vi "VI Tree.vi"   [LabVIEW 2020]
uses:
  GPP.lvlib
panel:
  # "SEE DIAGRAM\nFOR VI TREE."
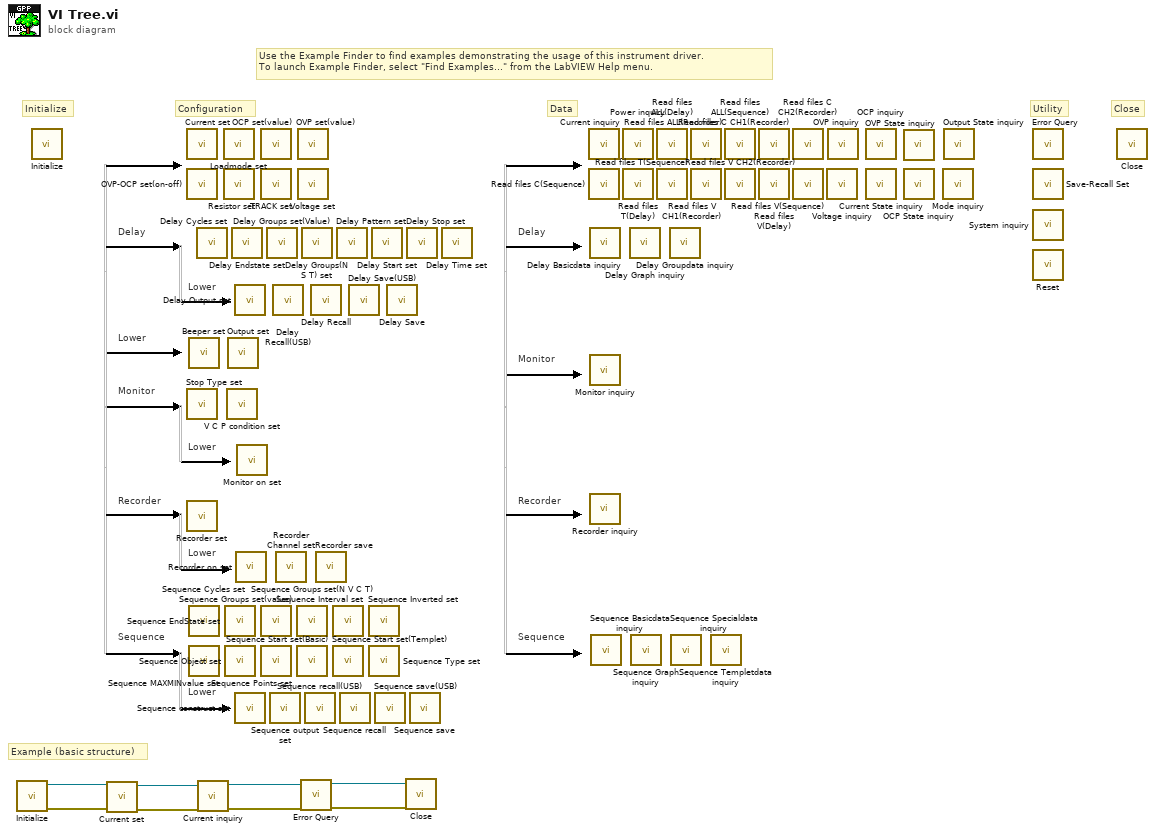
[diagram p0: block diagram]
diagram:
  # "Example (basic structure)"
  # "Sequence"
  # "Recorder"
  # "Monitor"
  # "Delay"
  # "Lower"
  # "Lower"
  # "Lower"
  # "Sequence"
  # "Recorder"
  # "Monitor"
  # "Lower"
  # "Lower"
  # "Delay"
  # "Configuration"
  # "Utility"
  # "Data"
  # "Close"
  # "Initialize"
  # "Use the Example Finder to find examples demonstrating the usage of this instrument driver.\nTo launch Example Finder, select \"Find Examples...\" from the LabVIEW Help menu."
  n1 = call "Initialize.vi"() -> ("error out"=w7:errorcluster, "VISA resource name out"=w8:refnum<visa-resource-name>)  [unwired: 9 in, 1 out]
  n2 = call "Initialize.vi"() -> ()  [unwired: 9 in, 3 out]
  n3 = call "Current set.vi"("error in (no error)"=w7, "VISA resource name"=w8) -> ("error out"=w5:errorcluster, "VISA resource name out"=w6:refnum<visa-resource-name>)  [unwired: 8 in]
  n4 = call "Current set.vi"() -> ()  [unwired: 10 in, 2 out]
  n5 = call "OVP-OCP set(on-off).vi"() -> ()  [unwired: 10 in, 2 out]
  n6 = call "Stop Type set.vi"() -> ()  [unwired: 10 in, 2 out]
  n7 = call "Recorder set.vi"() -> ()  [unwired: 10 in, 2 out]
  n8 = call "Beeper set.vi"() -> ()  [unwired: 10 in, 2 out]
  n9 = call "Sequence Cycles set.vi"() -> ()  [unwired: 10 in, 2 out]
  n10 = call "Sequence MAXMINvalue set.vi"() -> ()  [unwired: 10 in, 2 out]
  n11 = call "Delay Cycles set.vi"() -> ()  [unwired: 10 in, 2 out]
  n12 = call "Current inquiry.vi"("error in (no error)"=w5, "VISA resource name"=w6) -> ("error out"=w3:errorcluster, "VISA resource name out"=w4:refnum<visa-resource-name>)  [unwired: 7 in, 1 out]
  n13 = call "Loadmode set.vi"() -> ()  [unwired: 10 in, 2 out]
  n14 = call "Resistor set.vi"() -> ()  [unwired: 10 in, 2 out]
  n15 = call "Sequence EndState set.vi"() -> ()  [unwired: 10 in, 2 out]
  n16 = call "Sequence Object set.vi"() -> ()  [unwired: 10 in, 2 out]
  n17 = call "V C P condition set.vi"() -> ()  [unwired: 18 in, 2 out]
  n18 = call "Output set.vi"() -> ()  [unwired: 10 in, 2 out]
  n19 = call "Delay Endstate set.vi"() -> ()  [unwired: 10 in, 2 out]
  n20 = call "Delay Output set.vi"() -> ()  [unwired: 10 in, 2 out]
  n21 = call "Sequence construct set.vi"() -> ()  [unwired: 10 in, 2 out]
  n22 = call "Recorder on set.vi"() -> ()  [unwired: 10 in, 2 out]
  n23 = call "Monitor on set.vi"() -> ()  [unwired: 10 in, 2 out]
  n24 = call "OCP set(value).vi"() -> ()  [unwired: 10 in, 2 out]
  n25 = call "TRACK set.vi"() -> ()  [unwired: 10 in, 2 out]
  n26 = call "Sequence Groups set(value).vi"() -> ()  [unwired: 10 in, 2 out]
  n27 = call "Sequence Points set.vi"() -> ()  [unwired: 10 in, 2 out]
  n28 = call "Delay Groups set(Value).vi"() -> ()  [unwired: 10 in, 2 out]
  n29 = call "Sequence output set.vi"() -> ()  [unwired: 10 in, 2 out]
  n30 = call "Delay Recall(USB).vi"() -> ()  [unwired: 10 in, 2 out]
  n31 = call "Recorder Channel set.vi"() -> ()  [unwired: 10 in, 2 out]
  n32 = call "Sequence Groups set(N V C T).vi"() -> ()  [unwired: 10 in, 2 out]
  n33 = call "Sequence Start set(Basic).vi"() -> ()  [unwired: 10 in, 2 out]
  n34 = call "OVP set(value).vi"() -> ()  [unwired: 10 in, 2 out]
  n35 = call "Voltage set.vi"() -> ()  [unwired: 10 in, 2 out]
  n36 = call "Error Query.vi"("error in (no error)"=w3, "VISA resource name"=w4) -> ("error out"=w1:errorcluster, "VISA resource name out"=w2:refnum<visa-resource-name>)  [unwired: 6 in, 2 out]
  n37 = call "Delay Groups(N S T) set.vi"() -> ()  [unwired: 10 in, 2 out]
  n38 = call "Sequence recall(USB).vi"() -> ()  [unwired: 10 in, 2 out]
  n39 = call "Delay Recall.vi"() -> ()  [unwired: 10 in, 2 out]
  n40 = call "Recorder save.vi"() -> ()  [unwired: 10 in, 2 out]
  n41 = call "Sequence Interval set.vi"() -> ()  [unwired: 10 in, 2 out]
  n42 = call "Sequence Start set(Templet).vi"() -> ()  [unwired: 10 in, 2 out]
  n43 = call "Delay Pattern set.vi"() -> ()  [unwired: 10 in, 2 out]
  n44 = call "Sequence recall.vi"() -> ()  [unwired: 10 in, 2 out]
  n45 = call "Delay Save(USB).vi"() -> ()  [unwired: 10 in, 2 out]
  n46 = call "Sequence Inverted set.vi"() -> ()  [unwired: 10 in, 2 out]
  n47 = call "Sequence Type set.vi"() -> ()  [unwired: 10 in, 2 out]
  n48 = call "Delay Start set.vi"() -> ()  [unwired: 10 in, 2 out]
  n49 = call "Sequence save(USB).vi"() -> ()  [unwired: 10 in, 2 out]
  n50 = call "Delay Save.vi"() -> ()  [unwired: 10 in, 2 out]
  n51 = call "Close.vi"("error in (no error)"=w1, "VISA resource name"=w2) -> ()  [unwired: 9 in, 1 out]
  n52 = call "Delay Stop set.vi"() -> ()  [unwired: 10 in, 2 out]
  n53 = call "Sequence save.vi"() -> ()  [unwired: 10 in, 2 out]
  n54 = call "Delay Time set.vi"() -> ()  [unwired: 10 in, 2 out]
  n55 = call "Current inquiry.vi"() -> ()  [unwired: 9 in, 3 out]
  n56 = call "Read files C(Sequence).vi"() -> ()  [unwired: 11 in, 1 out]
  n57 = call "Delay Basicdata inquiry.vi"() -> ()  [unwired: 6 in, 6 out]
  n58 = call "Monitor inquiry.vi"() -> ()  [unwired: 7 in, 9 out]
  n59 = call "Recorder inquiry.vi"() -> ()  [unwired: 7 in, 5 out]
  n60 = call "Sequence Basicdata inquiry.vi"() -> ()  [unwired: 6 in, 6 out]
  n61 = call "Power inquiry.vi"() -> ()  [unwired: 9 in, 3 out]
  n62 = call "Read files T(Delay).vi"() -> ()  [unwired: 11 in, 1 out]
  n63 = call "Delay Graph inquiry.vi"() -> ()  [unwired: 12 in, 4 out]
  n64 = call "Sequence Graph inquiry.vi"() -> ()  [unwired: 12 in, 4 out]
  n65 = call "Read files ALL(Delay).vi"() -> ()  [unwired: 10 in, 2 out]
  n66 = call "Read files T(Sequence).vi"() -> ()  [unwired: 11 in, 1 out]
  n67 = call "Delay Groupdata inquiry.vi"() -> ()  [unwired: 8 in, 4 out]
  n68 = call "Sequence Specialdata inquiry.vi"() -> ()  [unwired: 6 in, 6 out]
  n69 = call "Read files ALL(Recorder).vi"() -> ()  [unwired: 8 in, 4 out]
  n70 = call "Read files V CH1(Recorder).vi"() -> ()  [unwired: 11 in, 1 out]
  n71 = call "Sequence Templetdata inquiry.vi"() -> ()  [unwired: 6 in, 10 out]
  n72 = call "Read files ALL(Sequence).vi"() -> ()  [unwired: 10 in, 2 out]
  n73 = call "Read files V CH2(Recorder).vi"() -> ()  [unwired: 11 in, 1 out]
  n74 = call "Read files C CH1(Recorder).vi"() -> ()  [unwired: 11 in, 1 out]
  n75 = call "Read files V(Delay).vi"() -> ()  [unwired: 11 in, 1 out]
  n76 = call "Read files C CH2(Recorder).vi"() -> ()  [unwired: 11 in, 1 out]
  n77 = call "Read files V(Sequence).vi"() -> ()  [unwired: 11 in, 1 out]
  n78 = call "Voltage inquiry.vi"() -> ()  [unwired: 9 in, 3 out]
  n79 = call "OVP inquiry.vi"() -> ()  [unwired: 9 in, 3 out]
  n80 = call "OCP inquiry.vi"() -> ()  [unwired: 9 in, 3 out]
  n81 = call "Current State inquiry.vi"() -> ()  [unwired: 9 in, 3 out]
  n82 = call "OVP State inquiry.vi"() -> ()  [unwired: 9 in, 3 out]
  n83 = call "OCP State inquiry.vi"() -> ()  [unwired: 9 in, 3 out]
  n84 = call "Mode inquiry.vi"() -> ()  [unwired: 9 in, 3 out]
  n85 = call "Output State inquiry.vi"() -> ()  [unwired: 9 in, 3 out]
  n86 = call "Error Query.vi"() -> ()  [unwired: 8 in, 4 out]
  n87 = call "Save-Recall Set.vi"() -> ()  [unwired: 10 in, 2 out]
  n88 = call "System inquiry.vi"() -> ()  [unwired: 8 in, 4 out]
  n89 = call "Reset.vi"() -> ()  [unwired: 10 in, 2 out]
  n90 = call "Close.vi"() -> ()  [unwired: 11 in, 1 out]
